vi "Create.vi"(8 "error in":errorcluster, 11 "Actor in":refnum<class "Actor.lvclass">) -> (0 "error out":errorcluster, 3 "Actor out":refnum<class "Actor.lvclass">)   [LabVIEW 2020, in "_Rescript.lvlib" / "Actor.lvlib" / "Actor.lvclass"]
uses:
  Actor.lvclass
  Actor.lvclass/Actor.ctl
  _Shared/Name Specs/Name Specs.lvclass
  _Shared/Project Stuff/Project Stuff.lvclass
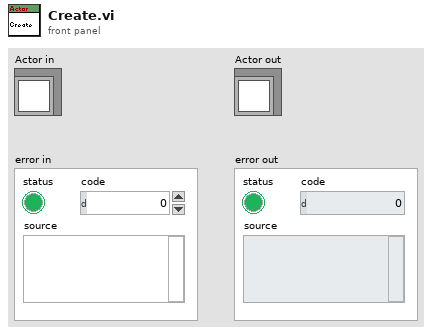
[diagram p1: front panel]
types:
  T1 = typedef "_Shared.lvlib/Name Stuff.ctl" = cluster{"Type (Enum)":T2, "Type (String)":string, "Name Library File Path":path, "Name":string, "Name Type":string}
  T2 = typedef "_Shared.lvlib/Type.ctl" = enum16{"Actor", "Msg"}
  T3 = typedef "_Rescript.lvlib/Actor.lvlib/Actor.lvclass/Name.ctl" = cluster{"Init Actor VI (Lib)":refnum<vi>}
  T4 = typedef "_Rescript.lvlib/Actor.lvlib/Actor.lvclass/Name Actor.ctl" = cluster{"Init Actor VI (Class)":refnum<vi>, "Init Actor VI (Lib)":refnum<vi>, "Terminal Attributes (Init)":T5}
  T5 = typedef "_Rescript.lvlib/Terminal Attributes.ctl" = map{i32, T6}
  T6 = typedef "_Rescript.lvlib/Attributes.ctl" = cluster{"Control":refnum<vi>, "Wire Rule":enum16{"Invalid Wire Rule", "Required", "Recommended", "Optional", "Dynamic Dispatch"}}
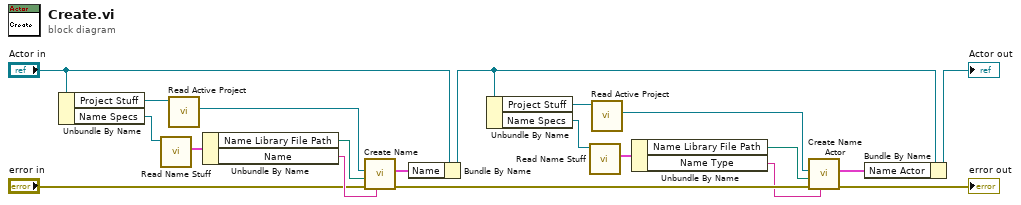
[diagram p0: block diagram]
diagram:
  n1 = Unbundle By Name("Actor in") -> ("Project Stuff"=w15:refnum<class "Project Stuff.lvclass">, "Name Specs"=w17:refnum<class "Name Specs.lvclass">)
  n2 = call "Read Name Stuff.vi"("Name Specs in"=w17) -> ("Name Stuff"=w16:T1)  [unwired: 10 in]
  n3 = call "Read Active Project.vi"("Project Stuff in"=w15) -> ("Active Project"=w11:refnum<vi>)  [unwired: 10 in]
  n4 = Unbundle By Name(w16) -> ("Name Library File Path"=w10:path, "Name"=w9:string)
  n5 = call "Create Name.vi"("Name"=w9, "error in"="error in", "Name Library File Path"=w10, "Active Project"=w11) -> ("error out"=w3:errorcluster, "Name"=w8:T3)  [unwired: 6 in]
  n6 = Bundle By Name(cluster="Actor in", "Name"=w8) -> (w14:refnum<class "Actor.lvclass">)
  n7 = Unbundle By Name(w14) -> ("Project Stuff"=w18:refnum<class "Project Stuff.lvclass">, "Name Specs"=w19:refnum<class "Name Specs.lvclass">)
  n8 = call "Read Name Stuff.vi"("Name Specs in"=w19) -> ("Name Stuff"=w20:T1)  [unwired: 10 in]
  n9 = call "Read Active Project.vi"("Project Stuff in"=w18) -> ("Active Project"=w7:refnum<vi>)  [unwired: 10 in]
  n10 = Unbundle By Name(w20) -> ("Name Library File Path"=w4:path, "Name Type"=w2:string)
  n11 = call "Create Name Actor.vi"("Name Actor"=w2, "error in"=w3, "Name Library File Path"=w4, "Active Project"=w7) -> ("error out"=→"error out":errorcluster, "Name Actor"=w1:T4)  [unwired: 6 in]
  n12 = Bundle By Name(cluster=w14, "Name Actor"=w1) -> (→"Actor out":refnum<class "Actor.lvclass">)
